vi "mrbraindetection1.vi"() -> ()   [LabVIEW 2017]
uses:
  <vilib>/vision/Image Controls.llb/IMAQ Image.ctl
  <vilib>/vision/NI_Vision_Development_Module.lvlib
panel:
  in  "Image Mask":T1
  in  "Image 2":T1
  in  "Thresholding range":cluster{"Lower value":sgl, "Upper value":sgl}={"Lower value"=128.0, "Upper value"=255.0} {"Upper value" format="%.2f"; "Lower value" format="%.2f"}
  out "error out":errorcluster
  out "Image":T1(plugin-control)
  out "Waveform Graph":T2(graph)
  in  "Interval Range 2":cluster{"Minimum":sgl, "Maximum":sgl} {"Maximum" format="%.2f"; "Minimum" format="%.2f"}
  out "Histogram Report":T3 {"Standard  Variation" format="%.2f"; "Mean Value" format="%.2f"; "Interval Width" format="%.2f"; "Starting Value" format="%.2f"; "Maximal Value" format="%.2f"; "Minimal Value" format="%.2f"}
  out "Mean Value":sgl format="%.2f"
  out "Standard  Deviation":sgl format="%.2f"
  in  "Interval Range":cluster{"Minimum":sgl, "Maximum":sgl} {"Maximum" format="%.2f"; "Minimum" format="%.2f"}
  out "File Type out":string
  in  "File Path":path
  out "File Data Type out":i32
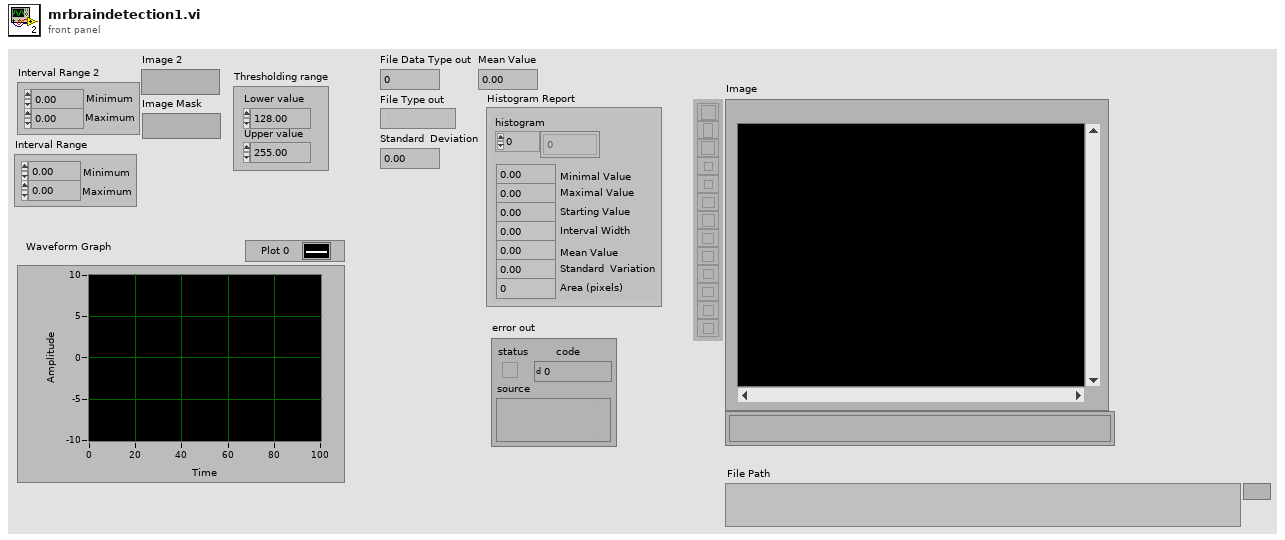
[diagram p1: front panel]
types:
  T1 = typedef "IMAQ Image.ctl" = refnum<image>
  T2 = cluster{"Starting Value":sgl, "Incremental Value":sgl, "Histogram":u32[]}
  T3 = cluster{"histogram":u32[], "Minimal Value":sgl, "Maximal Value":sgl, "Starting Value":sgl, "Interval Width":sgl, "Mean Value":sgl, "Standard  Variation":sgl, "Area (pixels)":i32}
  T4 = typedef "Image Type" = u32
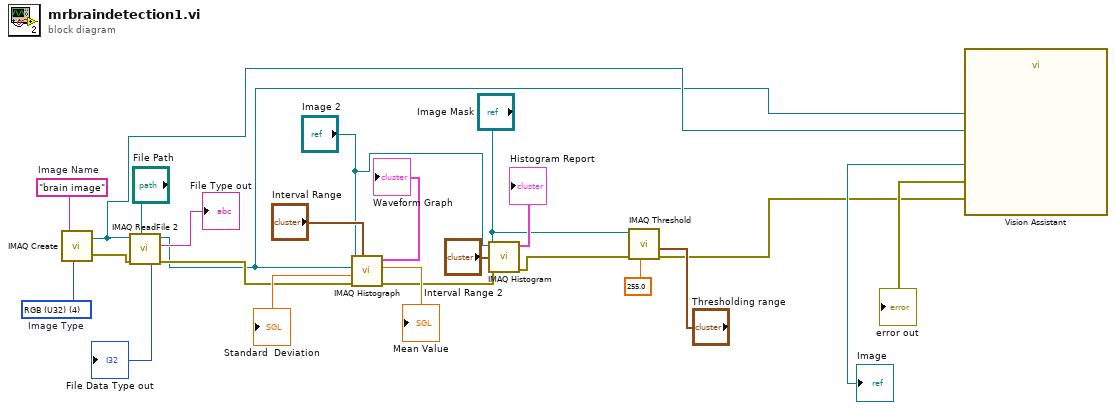
[diagram p0: block diagram]
diagram:
  w23 = T4 4 items=["Grayscale (U8)", "Grayscale (I16)", "Grayscale (SGL)", "Complex (CSG)", "RGB (U32)", "HSL (U32)", "RGB (U64)", "Grayscale (U16)"]  # Image Type
  w24 = "brain image"  # Image Name
  n1 = call "IMAQ Create"("Image Name"=w24, "Image Type"=w23) -> ("New Image"=w2:T1, "error out"=w6:errorcluster)  [unwired: 3 in]
  n2 = call "IMAQ ReadFile 2"("File Path"="File Path", "error in (no error)"=w6, "Image"=w2) -> ("error out"=w7:errorcluster, "File Data Type out"=→"File Data Type out":i32, "File Type out"=→"File Type out":string, "Image Out"=w1:T1)  [unwired: 4 in, 1 out]
  n3 = call "IMAQ Histograph"("error in (no error)"=w7, "Interval Range"="Interval Range", "Image Mask"=w1, "Image"="Image 2") -> ("error out"=w8:errorcluster, "Standard  Deviation"=→"Standard  Deviation":sgl, "Mean Value"=→"Mean Value":sgl, "Histogram Graph"=→"Waveform Graph":T2)  [unwired: 4 in]
  n4 = call "IMAQ Histogram"("error in (no error)"=w8, "Interval Range"="Interval Range 2", "Image Mask"="Image Mask", "Image"="Image 2") -> ("error out"=w10:errorcluster, "Histogram Report"=→"Histogram Report":T3)  [unwired: 6 in]
  n5 = call "IMAQ Threshold"("Replace Value"=sgl 255.0, "error in (no error)"=w10, "Range"="Thresholding range", "Image Src"="Image Mask") -> ("error out"=w9:errorcluster)  [unwired: 6 in, 1 out]
  n6 = call "Vision Assistant"("Image In"=w1, "Image Dst"=w2, "error in"=w9) -> ("Image Out"=→"Image":T1, "error out"=→"error out":errorcluster)  [unwired: 22 in, 1 out]
